vi "OCR Get Money.vi"(7 "error in":errorcluster, 10 "Path":path=path "C:/PokerSS/SS.png") -> (0 "error out":errorcluster, 3 "Player Money":string[](array[string]))   [LabVIEW 2015]
uses:
  <vilib>/vision/NI_Vision_Development_Module.lvlib
panel:
  out "Image Out":T1(plugin-control)
  out "String (Player10 Money)":string
  out "String (Player 9 Money)":string
  out "String (Player8 Money)":string
  out "String (Player7 Money)":string
  out "String (Player6 Money)":string
  out "String (Player5 Money)":string
  out "String (Player4 Money)":string
  out "String (Player3 Money)":string
  out "String (Player 2 Money)":string
  out "String (Player1 Money)":string
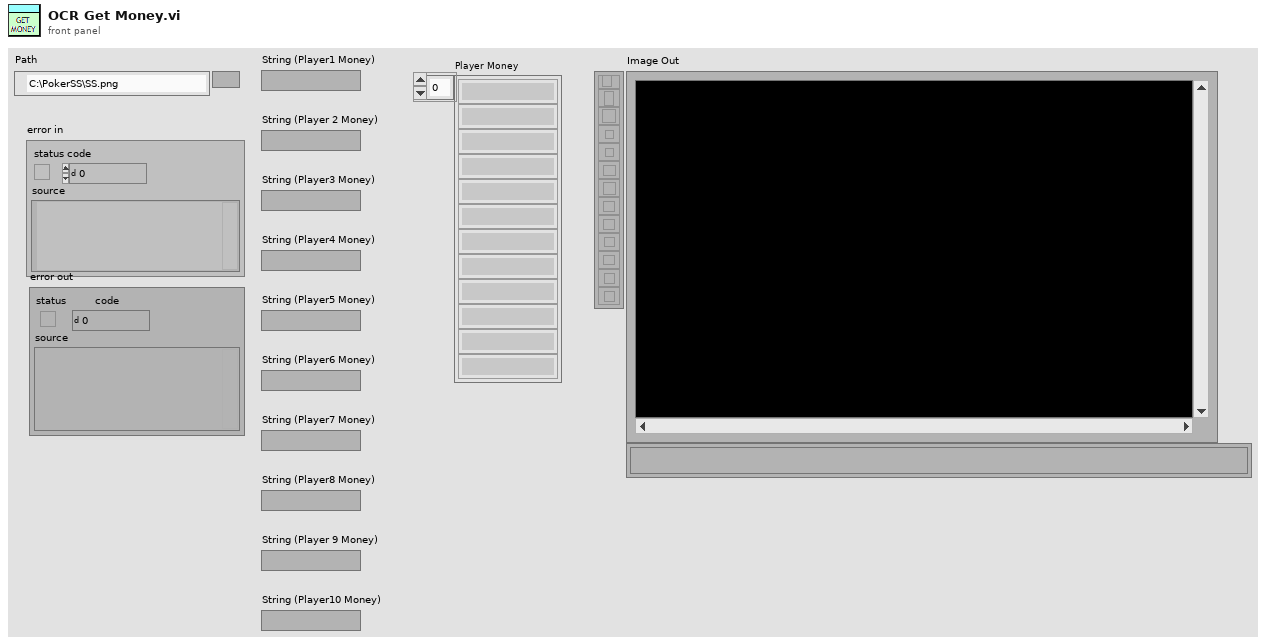
[diagram p1: front panel]
types:
  T1 = typedef "IMAQ Image.ctl" = refnum<image>
  T2 = cluster{"Threshold Data":cluster{"Method":enum16{"Fixed Range", "Uniform", "Linear", "Non Linear", "Local", "Color"}, "Looking for":u32, "Color Mode":u32, "Kernel Size":cluster{"Width":i32, "Height":i32}, "Ranges":cluster{"Min":i32, "Max":i32}[]}, "Reject Border":bool, "Number Of Erosions":i32, "Size & Spacing":cluster{"Segment Algorithm":u16, "Min Bounding Rect Width":i32, "Max Bounding Rect Width":i32, "Min Bounding Rect Height":i32, "Max Bounding Rect Height":i32, "Min Character Size":i32, "Max Character Size":i32, "Min Char Spacing":i32, "Max Horiz Element Spacing":i32, "Max Vert Element Spacing":i32, "Max Space Distance":i32}, "Read Options":cluster{"Read Strategy":i32, "Read Resolution":i32, "Scale Dependant":bool, "Aspect Ratio":i32, "Acceptance Level":i32, "Substitution Character":string, "MultiLine":bool}, "Valid Characters":cluster{"Pre-defined characters":i32, "User-defined characters":string}[], "Use Text Pattern":bool, "Orientation":u32, "# Lines Expected":u32, "Number of Blocks":i32}
  T3 = cluster{"Global Rectangle":i32[], "Contours":cluster{"ID":enum32{"External", "Internal"}, "Type":u32, "Coordinates":i32[]}[]}
  T4 = typedef "Image Type" = u32
  T5 = typedef "IMAQ OCR Session.ctl" = refnum<k1>
diagram:
  w27 = u32 0 items=["Grayscale", "Binary", "Gradient", "Rainbow", "Temperature", "User Defined", "Binary 16 Bit", "Gradient 16 Bit", "Rainbow 16 Bit", "Temperature 16 Bit", "User Defined 16 Bit"] ("Palette Type")
  w36 = T2 {"Threshold Data"={"Method"=enum."Uniform", "Looking for"=1, "Color Mode"=0, "Kernel Size"={"Width"=32, "Height"=32}, "Ranges"=[{"Min"=1, "Max"=255}]}, "Reject Border"=TRUE, "Number Of Erosions"=0, "Size & Spacing"={"Segment Algorithm"=0, "Min Bounding Rect Width"=2, "Max Bounding Rect Width"=8, "Min Bounding Rect Height"=2, "Max Bounding Rect Height"=65536, "Min Character Size"=4, "Max Character Size"=5555, "Min Char Spacing"=1, "Max Horiz Element Spacing"=1, "Max Vert Element Spacing"=0, "Max Space Distance"=65536}, "Read Options"={"Read Strategy"=1, "Read Resolution"=2, "Scale Dependant"=FALSE, "Aspect Ratio"=400, "Acceptance Level"=700, "Substitution Character"="?", "MultiLine"=FALSE}, "Valid Characters"=[], "Use Text Pattern"=FALSE, "Orientation"=0, "# Lines Expected"=0, "Number of Blocks"=4}  # Parameters
  w37 = T3 {"Global Rectangle"=[720, 494, 833, 511], "Contours"=[{"ID"=enum."External", "Type"=3, "Coordinates"=[720, 494, 833, 513]}]}  # ROI Descriptor
  w45 = T2 {"Threshold Data"={"Method"=enum."Uniform", "Looking for"=1, "Color Mode"=0, "Kernel Size"={"Width"=32, "Height"=32}, "Ranges"=[{"Min"=1, "Max"=255}]}, "Reject Border"=TRUE, "Number Of Erosions"=0, "Size & Spacing"={"Segment Algorithm"=0, "Min Bounding Rect Width"=2, "Max Bounding Rect Width"=8, "Min Bounding Rect Height"=2, "Max Bounding Rect Height"=65536, "Min Character Size"=4, "Max Character Size"=5555, "Min Char Spacing"=1, "Max Horiz Element Spacing"=1, "Max Vert Element Spacing"=0, "Max Space Distance"=65536}, "Read Options"={"Read Strategy"=1, "Read Resolution"=2, "Scale Dependant"=FALSE, "Aspect Ratio"=400, "Acceptance Level"=700, "Substitution Character"="?", "MultiLine"=FALSE}, "Valid Characters"=[], "Use Text Pattern"=FALSE, "Orientation"=0, "# Lines Expected"=0, "Number of Blocks"=4}  # Parameters
  w46 = T3 {"Global Rectangle"=[523, 533, 645, 550], "Contours"=[{"ID"=enum."External", "Type"=3, "Coordinates"=[523, 533, 645, 550]}]}  # ROI Descriptor
  w54 = T2 {"Threshold Data"={"Method"=enum."Uniform", "Looking for"=1, "Color Mode"=0, "Kernel Size"={"Width"=32, "Height"=32}, "Ranges"=[{"Min"=1, "Max"=255}]}, "Reject Border"=TRUE, "Number Of Erosions"=0, "Size & Spacing"={"Segment Algorithm"=0, "Min Bounding Rect Width"=2, "Max Bounding Rect Width"=8, "Min Bounding Rect Height"=2, "Max Bounding Rect Height"=65536, "Min Character Size"=4, "Max Character Size"=5555, "Min Char Spacing"=1, "Max Horiz Element Spacing"=1, "Max Vert Element Spacing"=0, "Max Space Distance"=65536}, "Read Options"={"Read Strategy"=1, "Read Resolution"=2, "Scale Dependant"=FALSE, "Aspect Ratio"=400, "Acceptance Level"=700, "Substitution Character"="?", "MultiLine"=FALSE}, "Valid Characters"=[], "Use Text Pattern"=FALSE, "Orientation"=0, "# Lines Expected"=0, "Number of Blocks"=4}  # Parameters
  w55 = T3 {"Global Rectangle"=[386, 689, 502, 706], "Contours"=[{"ID"=enum."External", "Type"=3, "Coordinates"=[386, 689, 502, 706]}]}  # ROI Descriptor
  w63 = T2 {"Threshold Data"={"Method"=enum."Uniform", "Looking for"=1, "Color Mode"=0, "Kernel Size"={"Width"=32, "Height"=32}, "Ranges"=[{"Min"=1, "Max"=255}]}, "Reject Border"=TRUE, "Number Of Erosions"=0, "Size & Spacing"={"Segment Algorithm"=0, "Min Bounding Rect Width"=2, "Max Bounding Rect Width"=8, "Min Bounding Rect Height"=2, "Max Bounding Rect Height"=65536, "Min Character Size"=4, "Max Character Size"=5555, "Min Char Spacing"=1, "Max Horiz Element Spacing"=1, "Max Vert Element Spacing"=0, "Max Space Distance"=65536}, "Read Options"={"Read Strategy"=1, "Read Resolution"=2, "Scale Dependant"=FALSE, "Aspect Ratio"=400, "Acceptance Level"=700, "Substitution Character"="?", "MultiLine"=FALSE}, "Valid Characters"=[], "Use Text Pattern"=FALSE, "Orientation"=0, "# Lines Expected"=0, "Number of Blocks"=4}  # Parameters
  w64 = T3 {"Global Rectangle"=[543, 836, 661, 852], "Contours"=[{"ID"=enum."External", "Type"=3, "Coordinates"=[543, 836, 661, 852]}]}  # ROI Descriptor
  w72 = T2 {"Threshold Data"={"Method"=enum."Uniform", "Looking for"=1, "Color Mode"=0, "Kernel Size"={"Width"=32, "Height"=32}, "Ranges"=[{"Min"=1, "Max"=255}]}, "Reject Border"=TRUE, "Number Of Erosions"=0, "Size & Spacing"={"Segment Algorithm"=0, "Min Bounding Rect Width"=2, "Max Bounding Rect Width"=8, "Min Bounding Rect Height"=2, "Max Bounding Rect Height"=65536, "Min Character Size"=4, "Max Character Size"=5555, "Min Char Spacing"=1, "Max Horiz Element Spacing"=1, "Max Vert Element Spacing"=0, "Max Space Distance"=65536}, "Read Options"={"Read Strategy"=1, "Read Resolution"=2, "Scale Dependant"=FALSE, "Aspect Ratio"=400, "Acceptance Level"=700, "Substitution Character"="?", "MultiLine"=FALSE}, "Valid Characters"=[], "Use Text Pattern"=FALSE, "Orientation"=0, "# Lines Expected"=0, "Number of Blocks"=4}  # Parameters
  w73 = T3 {"Global Rectangle"=[757, 870, 877, 886], "Contours"=[{"ID"=enum."External", "Type"=3, "Coordinates"=[757, 870, 877, 886]}]}  # ROI Descriptor
  w81 = T2 {"Threshold Data"={"Method"=enum."Uniform", "Looking for"=1, "Color Mode"=0, "Kernel Size"={"Width"=32, "Height"=32}, "Ranges"=[{"Min"=1, "Max"=255}]}, "Reject Border"=TRUE, "Number Of Erosions"=0, "Size & Spacing"={"Segment Algorithm"=0, "Min Bounding Rect Width"=2, "Max Bounding Rect Width"=8, "Min Bounding Rect Height"=2, "Max Bounding Rect Height"=65536, "Min Character Size"=4, "Max Character Size"=5555, "Min Char Spacing"=1, "Max Horiz Element Spacing"=1, "Max Vert Element Spacing"=0, "Max Space Distance"=65536}, "Read Options"={"Read Strategy"=1, "Read Resolution"=2, "Scale Dependant"=FALSE, "Aspect Ratio"=400, "Acceptance Level"=700, "Substitution Character"="?", "MultiLine"=FALSE}, "Valid Characters"=[], "Use Text Pattern"=FALSE, "Orientation"=0, "# Lines Expected"=0, "Number of Blocks"=4}  # Parameters
  w82 = T3 {"Global Rectangle"=[1029, 868, 1143, 888], "Contours"=[{"ID"=enum."External", "Type"=3, "Coordinates"=[1029, 868, 1143, 888]}]}  # ROI Descriptor
  w90 = T2 {"Threshold Data"={"Method"=enum."Uniform", "Looking for"=1, "Color Mode"=0, "Kernel Size"={"Width"=32, "Height"=32}, "Ranges"=[{"Min"=1, "Max"=255}]}, "Reject Border"=TRUE, "Number Of Erosions"=0, "Size & Spacing"={"Segment Algorithm"=0, "Min Bounding Rect Width"=2, "Max Bounding Rect Width"=8, "Min Bounding Rect Height"=2, "Max Bounding Rect Height"=65536, "Min Character Size"=4, "Max Character Size"=5555, "Min Char Spacing"=1, "Max Horiz Element Spacing"=1, "Max Vert Element Spacing"=0, "Max Space Distance"=65536}, "Read Options"={"Read Strategy"=1, "Read Resolution"=2, "Scale Dependant"=FALSE, "Aspect Ratio"=400, "Acceptance Level"=700, "Substitution Character"="?", "MultiLine"=FALSE}, "Valid Characters"=[], "Use Text Pattern"=FALSE, "Orientation"=0, "# Lines Expected"=0, "Number of Blocks"=4}  # Parameters
  w91 = T3 {"Global Rectangle"=[1264, 838, 1374, 853], "Contours"=[{"ID"=enum."External", "Type"=3, "Coordinates"=[1264, 838, 1374, 853]}]}  # ROI Descriptor
  w99 = T2 {"Threshold Data"={"Method"=enum."Uniform", "Looking for"=1, "Color Mode"=0, "Kernel Size"={"Width"=32, "Height"=32}, "Ranges"=[{"Min"=1, "Max"=255}]}, "Reject Border"=TRUE, "Number Of Erosions"=0, "Size & Spacing"={"Segment Algorithm"=0, "Min Bounding Rect Width"=2, "Max Bounding Rect Width"=8, "Min Bounding Rect Height"=2, "Max Bounding Rect Height"=65536, "Min Character Size"=4, "Max Character Size"=5555, "Min Char Spacing"=1, "Max Horiz Element Spacing"=1, "Max Vert Element Spacing"=0, "Max Space Distance"=65536}, "Read Options"={"Read Strategy"=1, "Read Resolution"=2, "Scale Dependant"=FALSE, "Aspect Ratio"=400, "Acceptance Level"=700, "Substitution Character"="?", "MultiLine"=FALSE}, "Valid Characters"=[], "Use Text Pattern"=FALSE, "Orientation"=0, "# Lines Expected"=0, "Number of Blocks"=4}  # Parameters
  w100 = T3 {"Global Rectangle"=[1385, 697, 1502, 712], "Contours"=[{"ID"=enum."External", "Type"=3, "Coordinates"=[1385, 697, 1502, 712]}]}  # ROI Descriptor
  w108 = T2 {"Threshold Data"={"Method"=enum."Uniform", "Looking for"=1, "Color Mode"=0, "Kernel Size"={"Width"=32, "Height"=32}, "Ranges"=[{"Min"=1, "Max"=255}]}, "Reject Border"=TRUE, "Number Of Erosions"=0, "Size & Spacing"={"Segment Algorithm"=0, "Min Bounding Rect Width"=2, "Max Bounding Rect Width"=8, "Min Bounding Rect Height"=2, "Max Bounding Rect Height"=65536, "Min Character Size"=4, "Max Character Size"=5555, "Min Char Spacing"=1, "Max Horiz Element Spacing"=1, "Max Vert Element Spacing"=0, "Max Space Distance"=65536}, "Read Options"={"Read Strategy"=1, "Read Resolution"=2, "Scale Dependant"=FALSE, "Aspect Ratio"=400, "Acceptance Level"=700, "Substitution Character"="?", "MultiLine"=FALSE}, "Valid Characters"=[], "Use Text Pattern"=FALSE, "Orientation"=0, "# Lines Expected"=0, "Number of Blocks"=4}  # Parameters
  w109 = T3 {"Global Rectangle"=[1253, 534, 1367, 552], "Contours"=[{"ID"=enum."External", "Type"=3, "Coordinates"=[1253, 534, 1367, 552]}]}  # ROI Descriptor
  w117 = T2 {"Threshold Data"={"Method"=enum."Uniform", "Looking for"=1, "Color Mode"=0, "Kernel Size"={"Width"=32, "Height"=32}, "Ranges"=[{"Min"=1, "Max"=255}]}, "Reject Border"=TRUE, "Number Of Erosions"=0, "Size & Spacing"={"Segment Algorithm"=0, "Min Bounding Rect Width"=2, "Max Bounding Rect Width"=8, "Min Bounding Rect Height"=2, "Max Bounding Rect Height"=65536, "Min Character Size"=4, "Max Character Size"=5555, "Min Char Spacing"=1, "Max Horiz Element Spacing"=1, "Max Vert Element Spacing"=0, "Max Space Distance"=65536}, "Read Options"={"Read Strategy"=1, "Read Resolution"=2, "Scale Dependant"=FALSE, "Aspect Ratio"=400, "Acceptance Level"=700, "Substitution Character"="?", "MultiLine"=FALSE}, "Valid Characters"=[], "Use Text Pattern"=FALSE, "Orientation"=0, "# Lines Expected"=0, "Number of Blocks"=4}  # Parameters
  w118 = T3 {"Global Rectangle"=[1068, 495, 1179, 514], "Contours"=[{"ID"=enum."External", "Type"=3, "Coordinates"=[1068, 495, 1179, 514]}]}  # ROI Descriptor
  w121 = 1 items=["Red", "Green", "Blue", "Hue", "Saturation", "Luminance", "Value", "Intensity"] ("Color Plane")
  w122 = T4 4 items=["Grayscale (U8)", "Grayscale (I16)", "Grayscale (SGL)", "Complex (CSG)", "RGB (U32)", "HSL (U32)", "RGB (U64)", "Grayscale (U16)"] ("Image Type")
  # "Was885"
  # "886 -> 888  SS3a"
  n1 = Call Chain() -> (call chain=w124:string[])
  n2 = Index Array(array=w124) -> (element=w123:string)  [unwired: 1 in]
  n3 = call "IMAQ Create"("Image Name"=w123, "Image Type"=w122, "error in (no error)"="error in") -> ("New Image"=w127:T1, "error out"=w126:errorcluster)  [unwired: 1 in, 1 out]
  n4 = call "IMAQ ReadFile"("File Path"="Path", "error in (no error)"=w126, "Image"=w127) -> ("error out"=w128:errorcluster, "Image Out"=w120:T1)  [unwired: 2 in, 5 out]
  n5 = call "IMAQ ExtractSingleColorPlane"("Color Plane"=w121, "error in (no error)"=w128, "Image Src"=w120) -> ("error out"=w119:errorcluster, "Image Dst Out"=w28:T1)  [unwired: 1 in, 6 out]
  "Image Out" <- w28
  n6 = while "Create an OCR session and read the character set file.\nSet paramaters from Vision Assistant Step." {
    shift-right: [w133] -> w115
    shift-left: _ -> [w132]
    tunnel: w119 -> [w135]
    tunnel: w117 -> [w131]
    tunnel: path "C:/Users/Bob Dabalina/Documents/Labview/Poker Hand2/Views Numbers.abc" ("File Path") -> [w130]
    tunnel: [w129] -> w116
    stop <- FALSE continue-if-true
    n7 = First Call?() -> (First Call?: T/F=w134:bool)
    n8 = case shown="True" w134 {
      tunnel: w130 -> [_ w142]
      tunnel: w135 -> [w137 w146]
      tunnel: [w138 w144] -> w133
      tunnel: [w137 w143] -> w129
      tunnel: w131 -> [_ w139]
      tunnel: w132 -> [w138 _]
      frame False {
      }
      frame True {
        w147 = 0 items=["Read All", "Read Character Set Only", "Read Properties Only"] ("Read Options")
        n9 = call <vilib>:"IVA Get Alternate Path.vi"("Path In"=w142) -> ("Path Out"=w141:path)  [unwired: 10 out]
        n10 = call "IMAQ OCR Create Session"("error in (no error)"=w146) -> ("error out"=w148:errorcluster, "IMAQ OCR Session"=w149:T5)  [unwired: 9 out]
        n11 = call "IMAQ OCR Read Character Set File"("File Path"=w141, "error in (no error)"=w148, "Read Options"=w147, "IMAQ OCR Session"=w149) -> ("error out"=w145:errorcluster, "IMAQ OCR Session (dup)"=w140:T5)  [unwired: 1 in, 5 out]
        n12 = call <vilib>:"IVA OCR - Set Parameters 2.vi"("error in (no error)"=w145, "Parameters"=w139, "IMAQ OCR Session"=w140) -> ("error out"=w143:errorcluster, "IMAQ OCR Session Out"=w144:T5)  [unwired: 7 in]
      }
    }
  }
  n13 = Unbundle By Name(w117) -> ("# Lines Expected"=w113:u32, "Orientation"=w114:u32)
  n14 = call "IMAQ OCR Read Text 4"("IMAQ OCR Session"=w115, "ROI Descriptor"=w118, "Image"=w28, "Number of Lines Requested"=w113, "error in (no error)"=w116, "Orientation"=w114) -> ("Read String"=w20:string, "error out"=w112:errorcluster)  [unwired: 8 out]
  "String (Player1 Money)" <- w20
  n15 = call <vilib>:"IVA Clear Coordsys Errors.vi"("error in (no error)"=w112) -> ("error out"=w111:errorcluster)  [unwired: 10 in]
  n16 = Initialize Array("", 0 ("dimension size")) -> (w21:string[])
  n17 = Insert Into Array(array=w21, index=0, new element=w20) -> (w19:string[])
  n18 = while "Create an OCR session and read the character set file.\nSet paramaters from Vision Assistant Step." {
    shift-right: [w154] -> w106
    shift-left: _ -> [w153]
    tunnel: w111 -> [w156]
    tunnel: w108 -> [w152]
    tunnel: path "C:/Users/Bob Dabalina/Documents/Labview/Poker Hand2/Views Numbers.abc" ("File Path") -> [w151]
    tunnel: [w150] -> w107
    stop <- FALSE continue-if-true
    n19 = First Call?() -> (First Call?: T/F=w155:bool)
    n20 = case shown="True" w155 {
      tunnel: w151 -> [_ w163]
      tunnel: w156 -> [w158 w167]
      tunnel: [w159 w165] -> w154
      tunnel: [w158 w164] -> w150
      tunnel: w152 -> [_ w160]
      tunnel: w153 -> [w159 _]
      frame False {
      }
      frame True {
        w168 = 0 items=["Read All", "Read Character Set Only", "Read Properties Only"] ("Read Options")
        n21 = call <vilib>:"IVA Get Alternate Path.vi"("Path In"=w163) -> ("Path Out"=w162:path)  [unwired: 10 out]
        n22 = call "IMAQ OCR Create Session"("error in (no error)"=w167) -> ("error out"=w169:errorcluster, "IMAQ OCR Session"=w170:T5)  [unwired: 9 out]
        n23 = call "IMAQ OCR Read Character Set File"("File Path"=w162, "error in (no error)"=w169, "Read Options"=w168, "IMAQ OCR Session"=w170) -> ("error out"=w166:errorcluster, "IMAQ OCR Session (dup)"=w161:T5)  [unwired: 1 in, 5 out]
        n24 = call <vilib>:"IVA OCR - Set Parameters 2.vi"("error in (no error)"=w166, "Parameters"=w160, "IMAQ OCR Session"=w161) -> ("error out"=w164:errorcluster, "IMAQ OCR Session Out"=w165:T5)  [unwired: 7 in]
      }
    }
  }
  n25 = Unbundle By Name(w108) -> ("# Lines Expected"=w104:u32, "Orientation"=w105:u32)
  n26 = call "IMAQ OCR Read Text 4"("IMAQ OCR Session"=w106, "ROI Descriptor"=w109, "Image"=w28, "Number of Lines Requested"=w104, "error in (no error)"=w107, "Orientation"=w105) -> ("Read String"=w18:string, "error out"=w103:errorcluster)  [unwired: 8 out]
  "String (Player 2 Money)" <- w18
  n27 = call <vilib>:"IVA Clear Coordsys Errors.vi"("error in (no error)"=w103) -> ("error out"=w102:errorcluster)  [unwired: 10 in]
  n28 = Build Array (concatenate)(w19, w18) -> (w17:string[])
  n29 = while "Create an OCR session and read the character set file.\nSet paramaters from Vision Assistant Step." {
    shift-right: [w175] -> w97
    shift-left: _ -> [w174]
    tunnel: w102 -> [w177]
    tunnel: w99 -> [w173]
    tunnel: path "C:/Users/Bob Dabalina/Documents/Labview/Poker Hand2/Views Numbers.abc" ("File Path") -> [w172]
    tunnel: [w171] -> w98
    stop <- FALSE continue-if-true
    n30 = First Call?() -> (First Call?: T/F=w176:bool)
    n31 = case shown="True" w176 {
      tunnel: w172 -> [_ w184]
      tunnel: w177 -> [w179 w188]
      tunnel: [w180 w186] -> w175
      tunnel: [w179 w185] -> w171
      tunnel: w173 -> [_ w181]
      tunnel: w174 -> [w180 _]
      frame False {
      }
      frame True {
        w189 = 0 items=["Read All", "Read Character Set Only", "Read Properties Only"] ("Read Options")
        n32 = call <vilib>:"IVA Get Alternate Path.vi"("Path In"=w184) -> ("Path Out"=w183:path)  [unwired: 10 out]
        n33 = call "IMAQ OCR Create Session"("error in (no error)"=w188) -> ("error out"=w190:errorcluster, "IMAQ OCR Session"=w191:T5)  [unwired: 9 out]
        n34 = call "IMAQ OCR Read Character Set File"("File Path"=w183, "error in (no error)"=w190, "Read Options"=w189, "IMAQ OCR Session"=w191) -> ("error out"=w187:errorcluster, "IMAQ OCR Session (dup)"=w182:T5)  [unwired: 1 in, 5 out]
        n35 = call <vilib>:"IVA OCR - Set Parameters 2.vi"("error in (no error)"=w187, "Parameters"=w181, "IMAQ OCR Session"=w182) -> ("error out"=w185:errorcluster, "IMAQ OCR Session Out"=w186:T5)  [unwired: 7 in]
      }
    }
  }
  n36 = Unbundle By Name(w99) -> ("# Lines Expected"=w95:u32, "Orientation"=w96:u32)
  n37 = call "IMAQ OCR Read Text 4"("IMAQ OCR Session"=w97, "ROI Descriptor"=w100, "Image"=w28, "Number of Lines Requested"=w95, "error in (no error)"=w98, "Orientation"=w96) -> ("Read String"=w16:string, "error out"=w94:errorcluster)  [unwired: 8 out]
  "String (Player3 Money)" <- w16
  n38 = call <vilib>:"IVA Clear Coordsys Errors.vi"("error in (no error)"=w94) -> ("error out"=w93:errorcluster)  [unwired: 10 in]
  n39 = Build Array (concatenate)(w17, w16) -> (w15:string[])
  n40 = while "Create an OCR session and read the character set file.\nSet paramaters from Vision Assistant Step." {
    shift-right: [w196] -> w88
    shift-left: _ -> [w195]
    tunnel: w93 -> [w198]
    tunnel: w90 -> [w194]
    tunnel: path "C:/Users/Bob Dabalina/Documents/Labview/Poker Hand2/Views Numbers.abc" ("File Path") -> [w193]
    tunnel: [w192] -> w89
    stop <- FALSE continue-if-true
    n41 = First Call?() -> (First Call?: T/F=w197:bool)
    n42 = case shown="True" w197 {
      tunnel: w193 -> [_ w205]
      tunnel: w198 -> [w200 w209]
      tunnel: [w201 w207] -> w196
      tunnel: [w200 w206] -> w192
      tunnel: w194 -> [_ w202]
      tunnel: w195 -> [w201 _]
      frame False {
      }
      frame True {
        w210 = 0 items=["Read All", "Read Character Set Only", "Read Properties Only"] ("Read Options")
        n43 = call <vilib>:"IVA Get Alternate Path.vi"("Path In"=w205) -> ("Path Out"=w204:path)  [unwired: 10 out]
        n44 = call "IMAQ OCR Create Session"("error in (no error)"=w209) -> ("error out"=w211:errorcluster, "IMAQ OCR Session"=w212:T5)  [unwired: 9 out]
        n45 = call "IMAQ OCR Read Character Set File"("File Path"=w204, "error in (no error)"=w211, "Read Options"=w210, "IMAQ OCR Session"=w212) -> ("error out"=w208:errorcluster, "IMAQ OCR Session (dup)"=w203:T5)  [unwired: 1 in, 5 out]
        n46 = call <vilib>:"IVA OCR - Set Parameters 2.vi"("error in (no error)"=w208, "Parameters"=w202, "IMAQ OCR Session"=w203) -> ("error out"=w206:errorcluster, "IMAQ OCR Session Out"=w207:T5)  [unwired: 7 in]
      }
    }
  }
  n47 = Unbundle By Name(w90) -> ("# Lines Expected"=w86:u32, "Orientation"=w87:u32)
  n48 = call "IMAQ OCR Read Text 4"("IMAQ OCR Session"=w88, "ROI Descriptor"=w91, "Image"=w28, "Number of Lines Requested"=w86, "error in (no error)"=w89, "Orientation"=w87) -> ("Read String"=w14:string, "error out"=w85:errorcluster)  [unwired: 8 out]
  "String (Player4 Money)" <- w14
  n49 = call <vilib>:"IVA Clear Coordsys Errors.vi"("error in (no error)"=w85) -> ("error out"=w84:errorcluster)  [unwired: 10 in]
  n50 = Build Array (concatenate)(w15, w14) -> (w13:string[])
  n51 = while "Create an OCR session and read the character set file.\nSet paramaters from Vision Assistant Step." {
    shift-right: [w217] -> w79
    shift-left: _ -> [w216]
    tunnel: w84 -> [w219]
    tunnel: w81 -> [w215]
    tunnel: path "C:/Users/Bob Dabalina/Documents/Labview/Poker Hand2/Views Numbers.abc" ("File Path") -> [w214]
    tunnel: [w213] -> w80
    stop <- FALSE continue-if-true
    n52 = First Call?() -> (First Call?: T/F=w218:bool)
    n53 = case shown="True" w218 {
      tunnel: w214 -> [_ w226]
      tunnel: w219 -> [w221 w230]
      tunnel: [w222 w228] -> w217
      tunnel: [w221 w227] -> w213
      tunnel: w215 -> [_ w223]
      tunnel: w216 -> [w222 _]
      frame False {
      }
      frame True {
        w231 = 0 items=["Read All", "Read Character Set Only", "Read Properties Only"] ("Read Options")
        n54 = call <vilib>:"IVA Get Alternate Path.vi"("Path In"=w226) -> ("Path Out"=w225:path)  [unwired: 10 out]
        n55 = call "IMAQ OCR Create Session"("error in (no error)"=w230) -> ("error out"=w232:errorcluster, "IMAQ OCR Session"=w233:T5)  [unwired: 9 out]
        n56 = call "IMAQ OCR Read Character Set File"("File Path"=w225, "error in (no error)"=w232, "Read Options"=w231, "IMAQ OCR Session"=w233) -> ("error out"=w229:errorcluster, "IMAQ OCR Session (dup)"=w224:T5)  [unwired: 1 in, 5 out]
        n57 = call <vilib>:"IVA OCR - Set Parameters 2.vi"("error in (no error)"=w229, "Parameters"=w223, "IMAQ OCR Session"=w224) -> ("error out"=w227:errorcluster, "IMAQ OCR Session Out"=w228:T5)  [unwired: 7 in]
      }
    }
  }
  n58 = Unbundle By Name(w81) -> ("# Lines Expected"=w77:u32, "Orientation"=w78:u32)
  n59 = call "IMAQ OCR Read Text 4"("IMAQ OCR Session"=w79, "ROI Descriptor"=w82, "Image"=w28, "Number of Lines Requested"=w77, "error in (no error)"=w80, "Orientation"=w78) -> ("Read String"=w12:string, "error out"=w76:errorcluster)  [unwired: 8 out]
  "String (Player5 Money)" <- w12
  n60 = call <vilib>:"IVA Clear Coordsys Errors.vi"("error in (no error)"=w76) -> ("error out"=w75:errorcluster)  [unwired: 10 in]
  n61 = Build Array (concatenate)(w13, w12) -> (w11:string[])
  n62 = while "Create an OCR session and read the character set file.\nSet paramaters from Vision Assistant Step." {
    shift-right: [w238] -> w70
    shift-left: _ -> [w237]
    tunnel: w75 -> [w240]
    tunnel: w72 -> [w236]
    tunnel: path "C:/Users/Bob Dabalina/Documents/Labview/Poker Hand2/Views Numbers.abc" ("File Path") -> [w235]
    tunnel: [w234] -> w71
    stop <- FALSE continue-if-true
    n63 = First Call?() -> (First Call?: T/F=w239:bool)
    n64 = case shown="True" w239 {
      tunnel: w235 -> [_ w247]
      tunnel: w240 -> [w242 w251]
      tunnel: [w243 w249] -> w238
      tunnel: [w242 w248] -> w234
      tunnel: w236 -> [_ w244]
      tunnel: w237 -> [w243 _]
      frame False {
      }
      frame True {
        w252 = 0 items=["Read All", "Read Character Set Only", "Read Properties Only"] ("Read Options")
        n65 = call <vilib>:"IVA Get Alternate Path.vi"("Path In"=w247) -> ("Path Out"=w246:path)  [unwired: 10 out]
        n66 = call "IMAQ OCR Create Session"("error in (no error)"=w251) -> ("error out"=w253:errorcluster, "IMAQ OCR Session"=w254:T5)  [unwired: 9 out]
        n67 = call "IMAQ OCR Read Character Set File"("File Path"=w246, "error in (no error)"=w253, "Read Options"=w252, "IMAQ OCR Session"=w254) -> ("error out"=w250:errorcluster, "IMAQ OCR Session (dup)"=w245:T5)  [unwired: 1 in, 5 out]
        n68 = call <vilib>:"IVA OCR - Set Parameters 2.vi"("error in (no error)"=w250, "Parameters"=w244, "IMAQ OCR Session"=w245) -> ("error out"=w248:errorcluster, "IMAQ OCR Session Out"=w249:T5)  [unwired: 7 in]
      }
    }
  }
  n69 = Unbundle By Name(w72) -> ("# Lines Expected"=w68:u32, "Orientation"=w69:u32)
  n70 = call "IMAQ OCR Read Text 4"("IMAQ OCR Session"=w70, "ROI Descriptor"=w73, "Image"=w28, "Number of Lines Requested"=w68, "error in (no error)"=w71, "Orientation"=w69) -> ("Read String"=w10:string, "error out"=w67:errorcluster)  [unwired: 8 out]
  "String (Player6 Money)" <- w10
  n71 = call <vilib>:"IVA Clear Coordsys Errors.vi"("error in (no error)"=w67) -> ("error out"=w66:errorcluster)  [unwired: 10 in]
  n72 = Build Array (concatenate)(w11, w10) -> (w9:string[])
  n73 = while "Create an OCR session and read the character set file.\nSet paramaters from Vision Assistant Step." {
    shift-right: [w259] -> w61
    shift-left: _ -> [w258]
    tunnel: w66 -> [w261]
    tunnel: w63 -> [w257]
    tunnel: path "C:/Users/Bob Dabalina/Documents/Labview/Poker Hand2/Views Numbers.abc" ("File Path") -> [w256]
    tunnel: [w255] -> w62
    stop <- FALSE continue-if-true
    n74 = First Call?() -> (First Call?: T/F=w260:bool)
    n75 = case shown="True" w260 {
      tunnel: w256 -> [_ w268]
      tunnel: w261 -> [w263 w272]
      tunnel: [w264 w270] -> w259
      tunnel: [w263 w269] -> w255
      tunnel: w257 -> [_ w265]
      tunnel: w258 -> [w264 _]
      frame False {
      }
      frame True {
        w273 = 0 items=["Read All", "Read Character Set Only", "Read Properties Only"] ("Read Options")
        n76 = call <vilib>:"IVA Get Alternate Path.vi"("Path In"=w268) -> ("Path Out"=w267:path)  [unwired: 10 out]
        n77 = call "IMAQ OCR Create Session"("error in (no error)"=w272) -> ("error out"=w274:errorcluster, "IMAQ OCR Session"=w275:T5)  [unwired: 9 out]
        n78 = call "IMAQ OCR Read Character Set File"("File Path"=w267, "error in (no error)"=w274, "Read Options"=w273, "IMAQ OCR Session"=w275) -> ("error out"=w271:errorcluster, "IMAQ OCR Session (dup)"=w266:T5)  [unwired: 1 in, 5 out]
        n79 = call <vilib>:"IVA OCR - Set Parameters 2.vi"("error in (no error)"=w271, "Parameters"=w265, "IMAQ OCR Session"=w266) -> ("error out"=w269:errorcluster, "IMAQ OCR Session Out"=w270:T5)  [unwired: 7 in]
      }
    }
  }
  n80 = Unbundle By Name(w63) -> ("# Lines Expected"=w59:u32, "Orientation"=w60:u32)
  n81 = call "IMAQ OCR Read Text 4"("IMAQ OCR Session"=w61, "ROI Descriptor"=w64, "Image"=w28, "Number of Lines Requested"=w59, "error in (no error)"=w62, "Orientation"=w60) -> ("Read String"=w8:string, "error out"=w58:errorcluster)  [unwired: 8 out]
  "String (Player7 Money)" <- w8
  n82 = call <vilib>:"IVA Clear Coordsys Errors.vi"("error in (no error)"=w58) -> ("error out"=w57:errorcluster)  [unwired: 10 in]
  n83 = Build Array (concatenate)(w9, w8) -> (w7:string[])
  n84 = while "Create an OCR session and read the character set file.\nSet paramaters from Vision Assistant Step." {
    shift-right: [w280] -> w52
    shift-left: _ -> [w279]
    tunnel: w57 -> [w282]
    tunnel: w54 -> [w278]
    tunnel: path "C:/Users/Bob Dabalina/Documents/Labview/Poker Hand2/Views Numbers.abc" ("File Path") -> [w277]
    tunnel: [w276] -> w53
    stop <- FALSE continue-if-true
    n85 = First Call?() -> (First Call?: T/F=w281:bool)
    n86 = case shown="True" w281 {
      tunnel: w277 -> [_ w289]
      tunnel: w282 -> [w284 w293]
      tunnel: [w285 w291] -> w280
      tunnel: [w284 w290] -> w276
      tunnel: w278 -> [_ w286]
      tunnel: w279 -> [w285 _]
      frame False {
      }
      frame True {
        w294 = 0 items=["Read All", "Read Character Set Only", "Read Properties Only"] ("Read Options")
        n87 = call <vilib>:"IVA Get Alternate Path.vi"("Path In"=w289) -> ("Path Out"=w288:path)  [unwired: 10 out]
        n88 = call "IMAQ OCR Create Session"("error in (no error)"=w293) -> ("error out"=w295:errorcluster, "IMAQ OCR Session"=w296:T5)  [unwired: 9 out]
        n89 = call "IMAQ OCR Read Character Set File"("File Path"=w288, "error in (no error)"=w295, "Read Options"=w294, "IMAQ OCR Session"=w296) -> ("error out"=w292:errorcluster, "IMAQ OCR Session (dup)"=w287:T5)  [unwired: 1 in, 5 out]
        n90 = call <vilib>:"IVA OCR - Set Parameters 2.vi"("error in (no error)"=w292, "Parameters"=w286, "IMAQ OCR Session"=w287) -> ("error out"=w290:errorcluster, "IMAQ OCR Session Out"=w291:T5)  [unwired: 7 in]
      }
    }
  }
  n91 = Unbundle By Name(w54) -> ("# Lines Expected"=w50:u32, "Orientation"=w51:u32)
  n92 = call "IMAQ OCR Read Text 4"("IMAQ OCR Session"=w52, "ROI Descriptor"=w55, "Image"=w28, "Number of Lines Requested"=w50, "error in (no error)"=w53, "Orientation"=w51) -> ("Read String"=w6:string, "error out"=w49:errorcluster)  [unwired: 8 out]
  "String (Player8 Money)" <- w6
  n93 = call <vilib>:"IVA Clear Coordsys Errors.vi"("error in (no error)"=w49) -> ("error out"=w48:errorcluster)  [unwired: 10 in]
  n94 = Build Array (concatenate)(w7, w6) -> (w5:string[])
  n95 = while "Create an OCR session and read the character set file.\nSet paramaters from Vision Assistant Step." {
    shift-right: [w301] -> w43
    shift-left: _ -> [w300]
    tunnel: w48 -> [w303]
    tunnel: w45 -> [w299]
    tunnel: path "C:/Users/Bob Dabalina/Documents/Labview/Poker Hand2/Views Numbers.abc" ("File Path") -> [w298]
    tunnel: [w297] -> w44
    stop <- FALSE continue-if-true
    n96 = First Call?() -> (First Call?: T/F=w302:bool)
    n97 = case shown="True" w302 {
      tunnel: w298 -> [_ w310]
      tunnel: w303 -> [w305 w314]
      tunnel: [w306 w312] -> w301
      tunnel: [w305 w311] -> w297
      tunnel: w299 -> [_ w307]
      tunnel: w300 -> [w306 _]
      frame False {
      }
      frame True {
        w315 = 0 items=["Read All", "Read Character Set Only", "Read Properties Only"] ("Read Options")
        n98 = call <vilib>:"IVA Get Alternate Path.vi"("Path In"=w310) -> ("Path Out"=w309:path)  [unwired: 10 out]
        n99 = call "IMAQ OCR Create Session"("error in (no error)"=w314) -> ("error out"=w316:errorcluster, "IMAQ OCR Session"=w317:T5)  [unwired: 9 out]
        n100 = call "IMAQ OCR Read Character Set File"("File Path"=w309, "error in (no error)"=w316, "Read Options"=w315, "IMAQ OCR Session"=w317) -> ("error out"=w313:errorcluster, "IMAQ OCR Session (dup)"=w308:T5)  [unwired: 1 in, 5 out]
        n101 = call <vilib>:"IVA OCR - Set Parameters 2.vi"("error in (no error)"=w313, "Parameters"=w307, "IMAQ OCR Session"=w308) -> ("error out"=w311:errorcluster, "IMAQ OCR Session Out"=w312:T5)  [unwired: 7 in]
      }
    }
  }
  n102 = Unbundle By Name(w45) -> ("# Lines Expected"=w41:u32, "Orientation"=w42:u32)
  n103 = call "IMAQ OCR Read Text 4"("IMAQ OCR Session"=w43, "ROI Descriptor"=w46, "Image"=w28, "Number of Lines Requested"=w41, "error in (no error)"=w44, "Orientation"=w42) -> ("Read String"=w4:string, "error out"=w40:errorcluster)  [unwired: 8 out]
  "String (Player 9 Money)" <- w4
  n104 = call <vilib>:"IVA Clear Coordsys Errors.vi"("error in (no error)"=w40) -> ("error out"=w39:errorcluster)  [unwired: 10 in]
  n105 = Build Array (concatenate)(w5, w4) -> (w3:string[])
  n106 = while "Create an OCR session and read the character set file.\nSet paramaters from Vision Assistant Step." {
    shift-right: [w322] -> w34
    shift-left: _ -> [w321]
    tunnel: w39 -> [w324]
    tunnel: w36 -> [w320]
    tunnel: path "C:/Users/Bob Dabalina/Documents/Labview/Poker Hand2/Views Numbers.abc" ("File Path") -> [w319]
    tunnel: [w318] -> w35
    stop <- FALSE continue-if-true
    n107 = First Call?() -> (First Call?: T/F=w323:bool)
    n108 = case shown="True" w323 {
      tunnel: w319 -> [_ w331]
      tunnel: w324 -> [w326 w335]
      tunnel: [w327 w333] -> w322
      tunnel: [w326 w332] -> w318
      tunnel: w320 -> [_ w328]
      tunnel: w321 -> [w327 _]
      frame False {
      }
      frame True {
        w336 = 0 items=["Read All", "Read Character Set Only", "Read Properties Only"] ("Read Options")
        n109 = call <vilib>:"IVA Get Alternate Path.vi"("Path In"=w331) -> ("Path Out"=w330:path)  [unwired: 10 out]
        n110 = call "IMAQ OCR Create Session"("error in (no error)"=w335) -> ("error out"=w337:errorcluster, "IMAQ OCR Session"=w338:T5)  [unwired: 9 out]
        n111 = call "IMAQ OCR Read Character Set File"("File Path"=w330, "error in (no error)"=w337, "Read Options"=w336, "IMAQ OCR Session"=w338) -> ("error out"=w334:errorcluster, "IMAQ OCR Session (dup)"=w329:T5)  [unwired: 1 in, 5 out]
        n112 = call <vilib>:"IVA OCR - Set Parameters 2.vi"("error in (no error)"=w334, "Parameters"=w328, "IMAQ OCR Session"=w329) -> ("error out"=w332:errorcluster, "IMAQ OCR Session Out"=w333:T5)  [unwired: 7 in]
      }
    }
  }
  n113 = Unbundle By Name(w36) -> ("# Lines Expected"=w32:u32, "Orientation"=w33:u32)
  n114 = call "IMAQ OCR Read Text 4"("IMAQ OCR Session"=w34, "ROI Descriptor"=w37, "Image"=w28, "Number of Lines Requested"=w32, "error in (no error)"=w35, "Orientation"=w33) -> ("Read String"=w26:string, "error out"=w31:errorcluster)  [unwired: 8 out]
  "String (Player10 Money)" <- w26
  n115 = call <vilib>:"IVA Clear Coordsys Errors.vi"("error in (no error)"=w31) -> ("error out"=w30:errorcluster)  [unwired: 10 in]
  n116 = property on="Image Out" class="ImageControl"(error in=w30, "Palette:Palette Type"=w27) -> (error out=→"error out":errorcluster)  [unwired: 1 in, 1 out]
  n117 = Build Array (concatenate)(w3, w26) -> (→"Player Money":string[])
